vi "Read UDP Connection .vi"(8 "error in (no error)":errorcluster, 11 "ReceiverState in":refnum<class "Connect Command.lvclass">) -> (0 "error out":errorcluster, 2 "UDP Connection":refnum<k16>, 3 "ReceiverState out":refnum<class "Connect Command.lvclass">)   [LabVIEW 2013, in "Receiver.lvlib" / "Receive Commands Using State Actors.lvlib" / "Connect Command.lvlib" / "Connect Command.lvclass"]
uses:
  Connect Command/Connect Command.lvclass
  Connect Command/Connect Command.lvclass/Connect Command.ctl
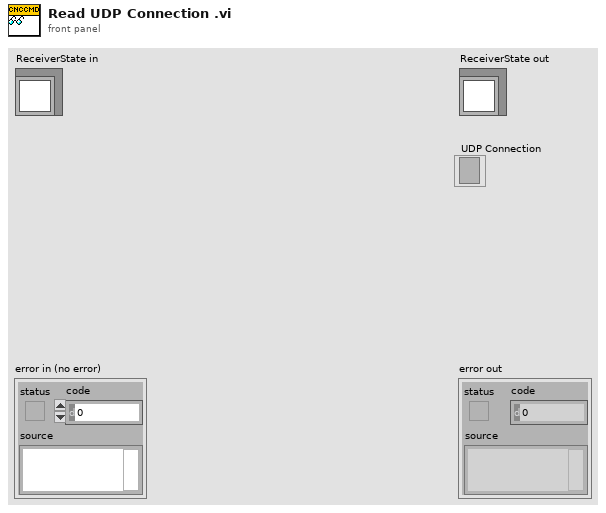
[diagram p1: front panel]
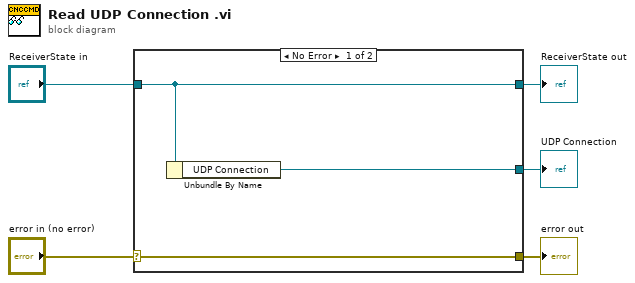
[diagram p0: block diagram]
diagram:
  n1 = case shown="No Error" "error in (no error)" {
    selector: "error in (no error)" -> [w8 w9]
    tunnel: [w8 w9] -> w4
    tunnel: [w7 w10] -> w2
    tunnel: "ReceiverState in" -> [w7 w10]
    tunnel: [w6 _] -> w1
    frame No Error {
      n2 = Unbundle By Name(w7) -> ("UDP Connection"=w6:refnum<k16>)
    }
    frame Error {
    }
  }
  "error out" <- w4
  "ReceiverState out" <- w2
  "UDP Connection" <- w1
